vi "Anomaly_Read_Dataset(as1D_refs).vi"(11 "sampling info":cluster{"Fs":dbl, "#s":dbl}={"Fs"=10000.0, "#s"=2000.0}) -> (0 "error out":errorcluster, 3 "DataSets_All(In1D_Out1D)":T1={"Train"={"Inputs Ref."=refnum, "Outputs Ref."=refnum, "Dims_In"=500, "Dataset_Size"=50000, "Dims_Out"=0, "Labels"=[], "File Paths"=[]}, "Validation"={"Inputs Ref."=refnum, "Outputs Ref."=refnum, "Dims_In"=500, "Dataset_Size"=100, "Dims_Out"=0, "Labels"=[], "File Paths"=[]}, "Test"={"Inputs Ref."=refnum, "Outputs Ref."=refnum, "Dims_In"=500, "Dataset_Size"=100, "Dims_Out"=0, "Labels"=[], "File Paths"=[]}})   [LabVIEW 2020]
uses:
  <vilib>/Ngene/DeepLTK/Toolkit/NN_Data/API/DataSet_Types/NN_DataSets_All(In1D_Out1D).ctl
  <vilib>/Ngene/DeepLTK/Toolkit/NN_Data/API/DataSet_Types/NN_DataSet(In1D_Out1D).ctl
  <vilib>/Ngene/DeepLTK/Toolkit/NN_Data/API/DataRef_Types/NN_Data_ref(2D_SGL).ctl
  <vilib>/Ngene/DeepLTK/Toolkit/NN_Data/subVIs/Dataset_Split/NN_DataSet_Split(In1D_Out1D).vi
  <vilib>/Ngene/DeepLTK/Toolkit/Deep_Learning_Toolkit_by_Ngene.lvlib
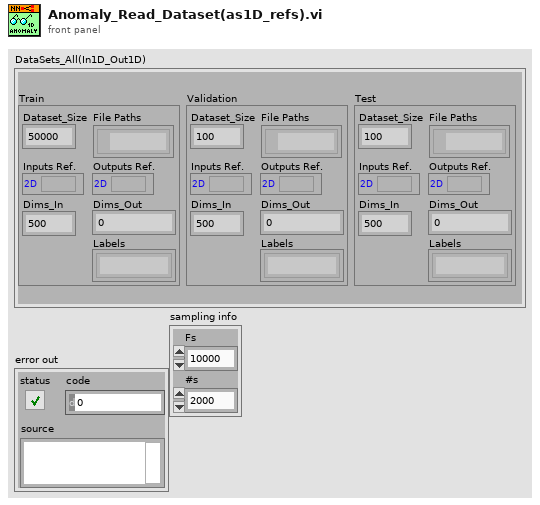
[diagram p1: front panel]
types:
  T1 = typedef "Deep_Learning_Toolkit_by_Ngene.lvlib/NN_DataSets_All(In1D_Out1D).ctl" = cluster{"Train":T2, "Validation":T2, "Test":T2}
  T2 = typedef "Deep_Learning_Toolkit_by_Ngene.lvlib/NN_DataSet(In1D_Out1D).ctl" = cluster{"Inputs Ref.":T3, "Outputs Ref.":T3, "Dims_In":i32, "Dataset_Size":i32, "Dims_Out":i32, "Labels":string[], "File Paths":path[]}
  T3 = typedef "Deep_Learning_Toolkit_by_Ngene.lvlib/NN_Data_ref(2D_SGL).ctl" = refnum<data-value>
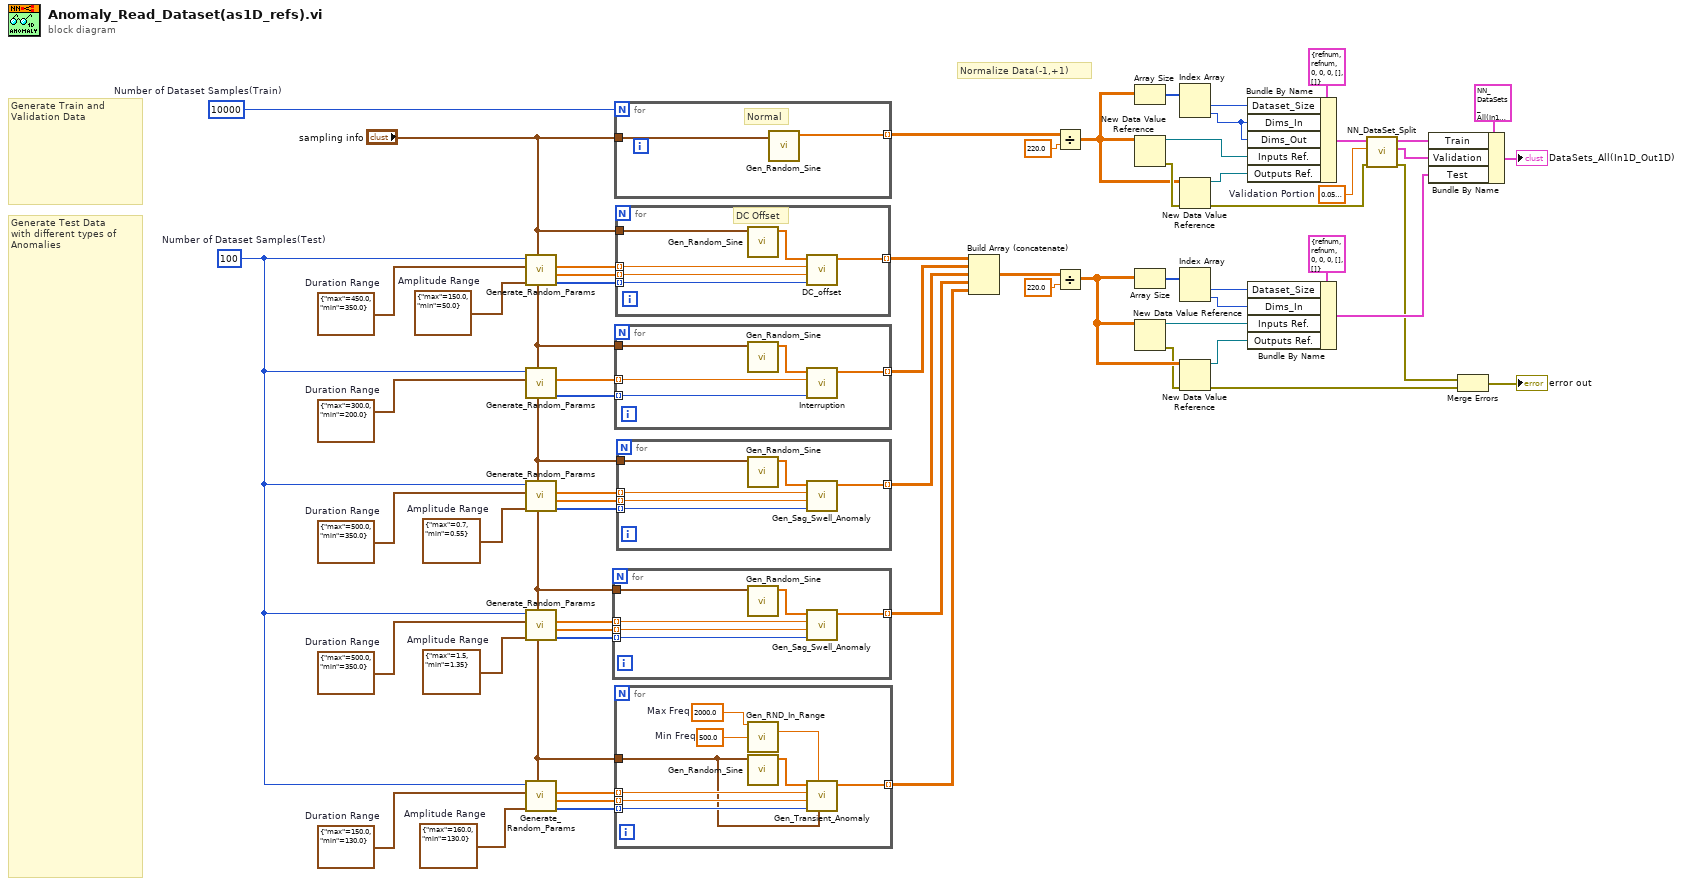
[diagram p0: block diagram]
diagram:
  w44 = sgl 0.05  # Validation Portion
  w35 = 10000  # Number of Dataset Samples(Train)
  w14 = cluster{"max":dbl, "min":dbl} {"max"=150.0, "min"=130.0}  # Duration Range
  w15 = cluster{"max":dbl, "min":dbl} {"max"=160.0, "min"=130.0}  # Amplitude Range
  w20 = cluster{"max":dbl, "min":dbl} {"max"=500.0, "min"=350.0}  # Duration Range
  w19 = cluster{"max":dbl, "min":dbl} {"max"=1.5, "min"=1.35}  # Amplitude Range
  w24 = cluster{"max":dbl, "min":dbl} {"max"=500.0, "min"=350.0}  # Duration Range
  w25 = cluster{"max":dbl, "min":dbl} {"max"=0.7, "min"=0.55}  # Amplitude Range
  w28 = cluster{"max":dbl, "min":dbl} {"max"=300.0, "min"=200.0}  # Duration Range
  w29 = cluster{"max":dbl, "min":dbl} {"max"=450.0, "min"=350.0}  # Duration Range
  w30 = cluster{"max":dbl, "min":dbl} {"max"=150.0, "min"=50.0}  # Amplitude Range
  w7 = 100  # Number of Dataset Samples(Test)
  # "Generate Test Data\nwith different types of Anomalies"
  # "Generate Train and Validation Data"
  # "Normalize Data(-1,+1)"
  n1 = call "Generate_Random_Params.vi"("sampling info"="sampling info", "Amplitude Range"=w30, "Duration Range"=w29, "Dataset Samples"=w7) -> ("Duration"=w31:i32[], "Amplitude"=w32:sgl[], "Position"=w33:dbl[])  [unwired: 5 in]
  n2 = call "Generate_Random_Params.vi"("sampling info"="sampling info", "Duration Range"=w28, "Dataset Samples"=w7) -> ("Duration"=w26:i32[], "Position"=w27:dbl[])  [unwired: 6 in, 1 out]
  n3 = call "Generate_Random_Params.vi"("sampling info"="sampling info", "Amplitude Range"=w25, "Duration Range"=w24, "Dataset Samples"=w7) -> ("Duration"=w21:i32[], "Amplitude"=w22:sgl[], "Position"=w23:dbl[])  [unwired: 5 in]
  n4 = call "Generate_Random_Params.vi"("sampling info"="sampling info", "Amplitude Range"=w19, "Duration Range"=w20, "Dataset Samples"=w7) -> ("Duration"=w16:i32[], "Amplitude"=w17:sgl[], "Position"=w18:dbl[])  [unwired: 5 in]
  n5 = call "Generate_Random_Params.vi"("sampling info"="sampling info", "Amplitude Range"=w15, "Duration Range"=w14, "Dataset Samples"=w7) -> ("Duration"=w11:i32[], "Amplitude"=w12:sgl[], "Position"=w13:dbl[])  [unwired: 5 in]
  n6 = for {
    tunnel: [w67] -> w3 mode=indexing
    tunnel: w18 -> [w66] mode=indexing
    tunnel: w17 -> [w65] mode=indexing
    tunnel: w16 -> [w64] mode=indexing
    tunnel: "sampling info" -> [w63]
    n7 = call "Gen_Random_Sine.vi"("sampling info"=w63) -> ("data"=w68:sgl[])  [unwired: 10 in]
    n8 = call "Gen_Sag_Swell_Anomaly.vi"("Duration"=w64, "Amplitude"=w65, "Position"=w66, "Sine"=w68) -> ("Sine+Anomaly"=w67:sgl[])  [unwired: 7 in]
  }
  n9 = for {
    N: w35 -> [_]
    tunnel: [w70] -> w4 mode=indexing
    tunnel: "sampling info" -> [w69]
    # "Normal"
    n10 = call "Gen_Random_Sine.vi"("sampling info"=w69) -> ("data"=w70:sgl[])  [unwired: 10 in]
  }
  n11 = for {
    tunnel: [w75] -> w9 mode=indexing
    tunnel: w27 -> [w73] mode=indexing
    tunnel: w26 -> [w72] mode=indexing
    tunnel: "sampling info" -> [w71]
    n12 = call "Gen_Random_Sine.vi"("sampling info"=w71) -> ("data"=w74:sgl[])  [unwired: 10 in]
    n13 = call "Interruption.vi"("Duration"=w72, "Position"=w73, "Sine"=w74) -> ("Sine+Anomaly"=w75:sgl[])  [unwired: 8 in]
  }
  n14 = for {
    tunnel: [w83] -> w8 mode=indexing
    tunnel: w13 -> [w79] mode=indexing
    tunnel: w12 -> [w78] mode=indexing
    tunnel: w11 -> [w77] mode=indexing
    tunnel: "sampling info" -> [w76]
    w80 = 2000.0  # Max Freq
    w81 = 500.0  # Min Freq
    n15 = call "Gen_RND_In_Range.vi"("Upper Bound"=w80, "Lower Bound"=w81) -> ("RND_In_Range"=w82:dbl)  [unwired: 13 in]
    n16 = call "Gen_Random_Sine.vi"("sampling info"=w76) -> ("data"=w84:sgl[])  [unwired: 10 in]
    n17 = call "Gen_Transient_Anomaly.vi"("sampling info"=w76, "Frequency"=w82, "Tau"=w77, "Amplitude"=w78, "Position"=w79, "Sine"=w84) -> ("Sine+Anomaly"=w83:sgl[])  [unwired: 5 in]
  }
  n18 = for {
    tunnel: [w89] -> w10 mode=indexing
    tunnel: w33 -> [w88] mode=indexing
    tunnel: w32 -> [w87] mode=indexing
    tunnel: w31 -> [w86] mode=indexing
    tunnel: "sampling info" -> [w85]
    # "DC Offset"
    n19 = call "Gen_Random_Sine.vi"("sampling info"=w85) -> ("data"=w90:sgl[])  [unwired: 10 in]
    n20 = call "DC_offset.vi"("Duration"=w86, "Ampltude"=w87, "Position"=w88, "Sine"=w90) -> ("Sine+Anomaly"=w89:sgl[])  [unwired: 7 in]
  }
  n21 = for {
    tunnel: [w95] -> w6 mode=indexing
    tunnel: w23 -> [w94] mode=indexing
    tunnel: w22 -> [w93] mode=indexing
    tunnel: w21 -> [w92] mode=indexing
    tunnel: "sampling info" -> [w91]
    n22 = call "Gen_Random_Sine.vi"("sampling info"=w91) -> ("data"=w96:sgl[])  [unwired: 10 in]
    n23 = call "Gen_Sag_Swell_Anomaly.vi"("Duration"=w92, "Amplitude"=w93, "Position"=w94, "Sine"=w96) -> ("Sine+Anomaly"=w95:sgl[])  [unwired: 7 in]
  }
  n24 = Build Array (concatenate)(w10, w9, w6, w3, w8) -> (w5:sgl[][])
  n25 = Divide(x=w4, y=sgl 220.0) -> (x/y=w34:sgl[][])
  n26 = Divide(x=w5, y=sgl 220.0) -> (x/y=w50:sgl[][])
  n27 = Array Size(array=w34) -> (size(s)=w60:i32[])
  n28 = New Data Value Reference(data value=w34) -> (data value reference=w62:refnum<data-value>, error out=w59:errorcluster)  [unwired: 1 in]
  n29 = Array Size(array=w50) -> (size(s)=w52:i32[])
  n30 = New Data Value Reference(data value=w50) -> (data value reference=w51:refnum<data-value>, error out=w43:errorcluster)  [unwired: 1 in]
  n31 = Index Array(array=w60) -> (element #1=w37:i32, element #2=w2:i32)  [unwired: 2 in]
  n32 = New Data Value Reference(data value=w34, error in=w59) -> (data value reference=w61:refnum<data-value>, error out=w42:errorcluster)
  n33 = Index Array(array=w52) -> (element #1=w53:i32, element #2=w54:i32)  [unwired: 2 in]
  n34 = New Data Value Reference(data value=w50, error in=w43) -> (data value reference=w49:refnum<data-value>, error out=w39:errorcluster)
  n35 = Bundle By Name(cluster=T2 {"Inputs Ref."=refnum, "Outputs Ref."=refnum, "Dims_In"=0, "Dataset_Size"=0, "Dims_Out"=0, "Labels"=[], "File Paths"=[]} ("Dataset(In1D_Out1D)"), "Dataset_Size"=w37, "Dims_In"=w2, "Dims_Out"=w2, "Inputs Ref."=w62, "Outputs Ref."=w61) -> (w47:T2)
  n36 = Bundle By Name(cluster=T2 {"Inputs Ref."=refnum, "Outputs Ref."=refnum, "Dims_In"=0, "Dataset_Size"=0, "Dims_Out"=0, "Labels"=[], "File Paths"=[]} ("Dataset(In1D_Out1D)"), "Dataset_Size"=w53, "Dims_In"=w54, "Inputs Ref."=w51, "Outputs Ref."=w49) -> (w48:T2)
  n37 = call-poly <vilib>:"NN_DataSet_Split.vi"("error in(no error)"=w42, "Split Size"=w44, "Dataset In"=w47) -> ("error out"=w41:errorcluster, "Dataset Out 2"=w45:T2, "Dataset Out 1"=w46:T2)  [unwired: 6 in]
  n38 = Bundle By Name(cluster=T1 {"Train"={"Inputs Ref."=refnum, "Outputs Ref."=refnum, "Dims_In"=0, "Dataset_Size"=0, "Dims_Out"=0, "Labels"=[], "File Paths"=[]}, "Validation"={"Inputs Ref."=refnum, "Outputs Ref."=refnum, "Dims_In"=0, "Dataset_Size"=0, "Dims_Out"=0, "Labels"=[], "File Paths"=[]}, "Test"={"Inputs Ref."=refnum, "Outputs Ref."=refnum, "Dims_In"=0, "Dataset_Size"=0, "Dims_Out"=0, "Labels"=[], "File Paths"=[]}} ("DataSets_All(In1D_Out1D)"), "Train"=w46, "Validation"=w45, "Test"=w48) -> (→"DataSets_All(In1D_Out1D)":T1)
  n39 = Merge Errors(w41, w39) -> (→"error out":errorcluster)
